vi "ap get board version string.vi"(9 "destLength":i32, 10 "BYTE_ARRAY":string, 11 "ap_handle":u32) -> (1 "function return":i32, 2 "BYTE_ARRAY out":string, 3 "ap_handle out":u32)   [LabVIEW 2019, in "apdm.lvlib"]
doc: "APDM_EXPORT int apdm_ap_get_board_version_string(apdm_ap_handle_t ap_handle, char *BYTE_ARRAY, const int destLength);"
uses:
  apdm.lvlib
  Lee Lab/CP FES Walking 2018/Code/Working/LabVIEW/apdm.dll
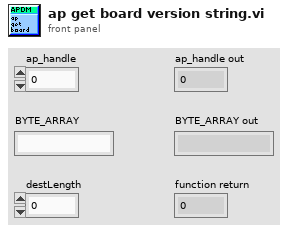
[diagram p1: front panel]
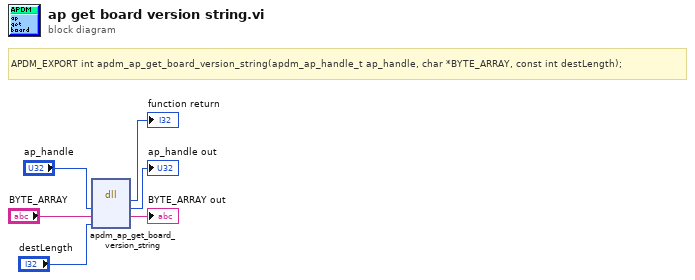
[diagram p0: block diagram]
diagram:
  # "APDM_EXPORT int apdm_ap_get_board_version_string(apdm_ap_handle_t ap_handle, char *BYTE_ARRAY, const int destLength);"
  n1 = dll-call lib="C:/Users/jfalesi/Dropbox/Lee Lab/CP FES Walking 2018/Code/Working/LabVIEW/apdm.*" fn="apdm_ap_get_board_version_string"("ap_handle"="ap_handle", "BYTE_ARRAY"="BYTE_ARRAY", "destLength"="destLength") -> (→"function return":i32, "ap_handle"=→"ap_handle out":u32, "BYTE_ARRAY"=→"BYTE_ARRAY out":string)  [unwired: 4 in, 2 out]
